vi "Test Neopixel Legacy.vi"() -> ()   [LabVIEW 2021]
uses:
  <vilib>/eio/EIONode/EIONode.xnode
  <vilib>/rvi/eio/common/nirviEmuTemplateMethod_errors.vi
  <vilib>/rvi/DataTransferAndStorage/Container/XNode/niFpgaContainer.xnode
  <vilib>/rvi/Memory/Memory_Emulation/nirvimemoryFastEmulation.vi
  <vilib>/rvi/Memory/Memory_Emulation/nirvimemoryEmulation.vi
  Public/Controls/Neopixel FIFO.ctl
  Neopixel - FPGA.lvlib
  <vilib>/rvi/FIFO/Fifo_Resource/niFpgaFifoEmulationRefIn.vi
panel:
  in  "Number Of Elements":i32=192
  in  "Update":bool
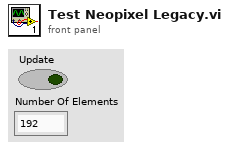
[diagram p1: front panel]
types:
  T1 = typedef "Neopixel - FPGA.lvlib/Neopixel FIFO.ctl" = refnum<k21>
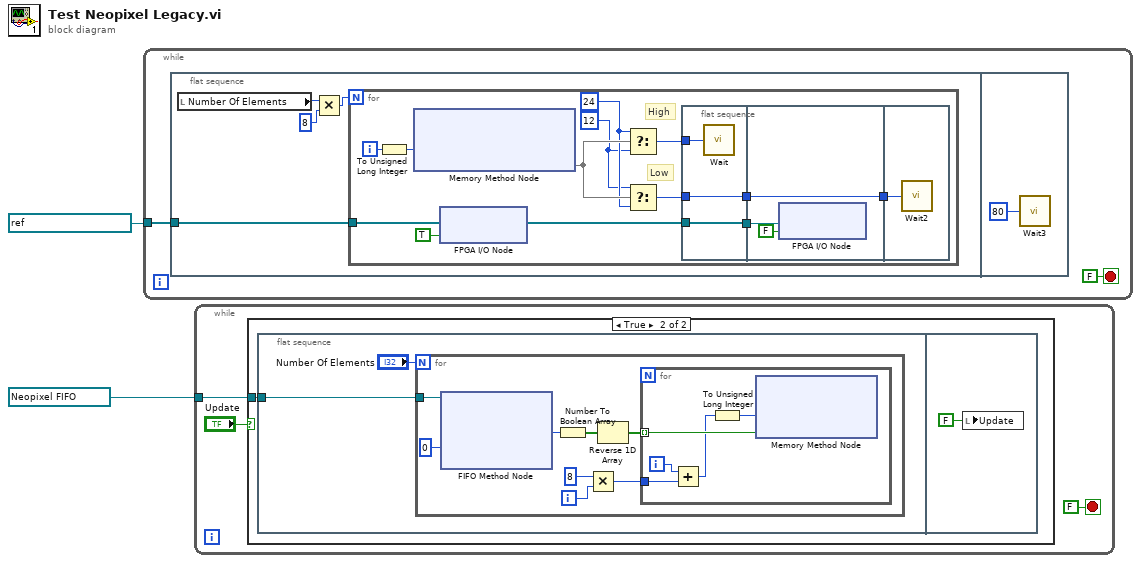
[diagram p0: block diagram]
diagram:
  n1 = while {
    tunnel: refnum<k21> "ConnectorC/DIO0" ("FPGA I/O In") -> [w3]
    stop <- FALSE stop-if-true
    n2 = flat-sequence {
      tunnel: w3 -> [w8]
      frame #0 {
        n3 = local read "Number Of Elements"() -> (w7:i32)
        n4 = Multiply(x=w7, y=8) -> (x*y=w5:i32)
        n5 = for {
          N: w5 -> [_]
          tunnel: w8 -> [w12]
          i -> [w20]
          w9 = u8 12 ("High False")
          w10 = u8 24 ("High True")
          # "Low"
          # "High"
          n6 = To Unsigned Long Integer(number=w20) -> (unsigned 32bit integer=w21:u32)
          n7 = xnode ("Memory Method Node")("Address"=w21) -> ("Data"=w17)  [unwired: 1 in, 1 out]
          n8 = xnode "FPGA I/O Node"("I/O Item"=TRUE, "FPGA I/O In"=w12) -> ("FPGA I/O Out"=w11:refnum<k21>)
          n9 = Select(t=w10, s=w17, f=w9) -> (s? t:f=w18:u8)
          n10 = Select(t=w9, s=w17, f=w10) -> (s? t:f=w16:u8)
          n11 = flat-sequence {
            tunnel: [w23] -> w19
            tunnel: [w24] -> w14
            tunnel: w16 -> [w24]
            tunnel: w18 -> [w22]
            tunnel: w11 -> [w23]
            tunnel: w19 -> [w27]
            tunnel: [w25] -> w15
            tunnel: w14 -> [w25]
            tunnel: w15 -> [w28]
            frame #0 {
              n12 = call "Wait"("Count(Ticks)"=w22) -> ()  [unwired: 1 out]
            }
            frame #1 {
              n13 = xnode "FPGA I/O Node"("I/O Item"=FALSE, "FPGA I/O In"=w27) -> ()  [unwired: 1 out]
            }
            frame #2 {
              n14 = call "Wait2"("Count(Ticks)"=w28) -> ()  [unwired: 1 out]
            }
          }
        }
      }
      frame #1 {
        n15 = call "Wait3"("Count(uSec)"=u16 80 ("Reset (us)")) -> ()  [unwired: 1 out]
      }
    }
  }
  n16 = while {
    tunnel: T1 "Neopixel FIFO" ("FIFO In") -> [w30]
    stop <- FALSE stop-if-true
    n17 = case shown="True" "Update" {
      tunnel: w30 -> [_ w33]
      frame False {
      }
      frame True {
        n18 = flat-sequence {
          tunnel: w33 -> [w35]
          frame #0 {
            n19 = for {
              N: "Number Of Elements" -> [_]
              tunnel: w35 -> [w37]
              i -> [w43]
              n20 = xnode ("FIFO Method Node")("Timeout"=0, "FIFO In"=w37) -> ("Element"=w38:u8)  [unwired: 2 out]
              n21 = Number To Boolean Array(number=w38) -> (Boolean array=w40:bool[])
              n22 = Multiply(x=8, y=w43) -> (x*y=w41:i32)
              n23 = Reverse 1D Array(array=w40) -> (reversed array=w39:bool[])
              n24 = for {
                tunnel: w39 -> [w47] mode=indexing
                tunnel: w41 -> [w45]
                i -> [w46]
                n25 = Add(x=w46, y=w45) -> (x+y=w44:i32)
                n26 = To Unsigned Long Integer(number=w44) -> (unsigned 32bit integer=w48:u32)
                n27 = xnode ("Memory Method Node")("Address"=w48, "Data"=w47) -> ()  [unwired: 1 in, 1 out]
              }
            }
          }
          frame #1 {
            n28 = local write "Update"(FALSE ("Update")) -> ()
          }
        }
      }
    }
  }
